vi "Stop Core.vi"(10 "final error code":i32, 11 "PersistantConnectionHandler in":refnum<class "PersistantConnectionHandler.lvclass">) -> (3 "PersistantConnectionHandler out":refnum<class "PersistantConnectionHandler.lvclass">)   [LabVIEW 2019, in "PersitantConnectionHandler.lvlib" / "PersistantConnectionHandler.lvclass"]
doc: "(<B>Filename</B>: Actor Framework.lvlib:Actor.lvclass:Stop Core.vi)\n\nDefines what the actor does before it stops. Use the <B>final error code</B> input to determine whether the actor shut down in response to an error.\n\nBy default, this method does nothing. A descendant class may override it to define behavior, such as shutting down any processes the actor initiated in its override of the Actor Core method."
uses:
  <vilib>/gpm_packages/@cs/Network-interface/Source/PersistantConnectionHandler/PersistantConnectionHandler/PersistantConnectionHandler.lvclass
  <vilib>/gpm_packages/@cs/Network-interface/Source/PersistantConnectionHandler/PersistantConnectionHandler/PersistantConnectionHandler.lvclass/PersistantConnectionHandler.ctl
  <vilib>/ActorFramework/Message Enqueuer/Message Enqueuer.lvclass/Message Enqueuer.ctl
  <vilib>/ActorFramework/Message Enqueuer/Enqueue.vi
  <vilib>/ActorFramework/Stop Msg/Stop Msg.lvclass
  C:/Program Files/National Instruments/LabVIEW 2019/vi.lib/ActorFramework/Message/Message.lvclass
  <vilib>/ActorFramework/Message Priority Queue/Priority Enqueue.vi
  <vilib>/gpm_packages/@cs/Network-interface/Source/Logged Actor/LoggedActor.lvclass
  <vilib>/gpm_packages/@cs/Network-interface/Source/MessagingInterfaces/IConnectionStateChangeCallback/IConnectionStateChangeCallback.lvclass
  <vilib>/gpm_packages/@cs/Network-interface/Source/Connection Factory Session/ConnectionFactorySession/ConnectionFactorySession.lvclass
  <vilib>/gpm_packages/@cs/Network-interface/Source/Connection Reference/Connection Reference/Connection Reference.lvclass
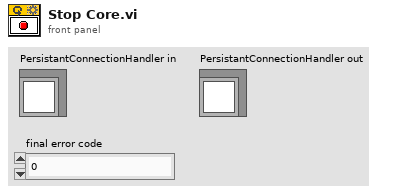
[diagram p1: front panel]
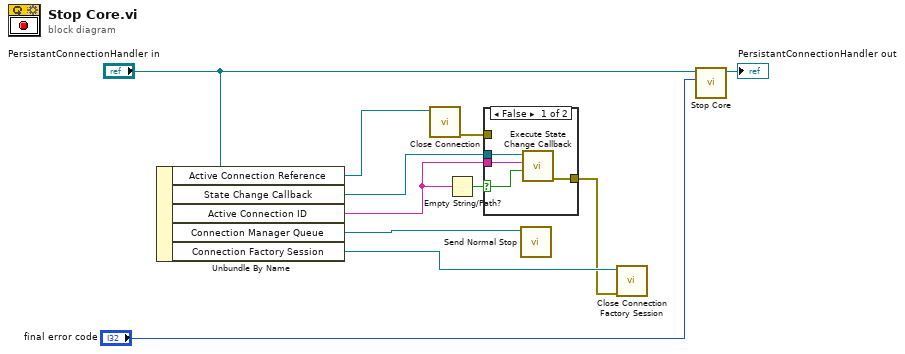
[diagram p0: block diagram]
diagram:
  n1 = Unbundle By Name("PersistantConnectionHandler in") -> ("Active Connection Reference"=w7:refnum<data-value>, "State Change Callback"=w6:refnum<class "IConnectionStateChangeCallback.lvclass">, "Active Connection ID"=w5:string, "Connection Manager Queue"=w8:refnum<class "Message Enqueuer.lvclass">, "Connection Factory Session"=w2:refnum<data-value>)
  n2 = call <vilib>:"Close Connection.vi"("Connection Reference In"=w7) -> ("error out"=w3:errorcluster)  [unwired: 10 in]
  n3 = Empty String/Path?(string/path=w5) -> (empty?=w4:bool)
  n4 = case shown="False" w4 {
    selector: w4 -> [w13 _]
    tunnel: w6 -> [w15 _]
    tunnel: w5 -> [w14 _]
    tunnel: w3 -> [_ _]
    tunnel: [w12 _] -> w1
    frame False {
      n5 = call-dynamic "Execute State Change Callback.vi"("Connection State"=w13, "Connection ID"=w14, "IConnectionStateChangeCallback in"=w15) -> ("error out"=w12:errorcluster)  [unwired: 8 in]
    }
    frame True {
    }
  }
  n6 = call <vilib>:"Send Normal Stop.vi"("Message Enqueuer"=w8) -> ()  [unwired: 10 in, 1 out]
  n7 = call <vilib>:"Close Connection Factory Session.vi"("error in (no error)"=w1, "Connection Factory Session In"=w2) -> ()  [unwired: 9 in, 1 out]
  n8 = call-parent "Stop Core.vi"("final error code"="final error code", "LoggedActor in"="PersistantConnectionHandler in") -> ("LoggedActor out"=→"PersistantConnectionHandler out":refnum<class "PersistantConnectionHandler.lvclass">)  [unwired: 9 in]
